vi "AIT 1553 - Parse RT Channels.vi"(6 "Bus Config Info":T10, 7 "FIFO Idx Qs":T12, 8 "error in (no error)":errorcluster, 9 "Bus Page Ref":T1 format="%.0x", 10 "Section GUID":string, 11 "Device Reference in":T1 format="%.0x") -> (0 "error out":errorcluster, 1 "Section BaseRate":u32, 2 "HW Channel - RT Section":T2 {"Message Settings"."Driver Data"."First Word" min=8 max=31; "Message Settings"."Driver Data"."Num Bits" min=1 max=32; "Message Settings"."Driver Data"."Start Bit" min=8 max=31; "Message Settings"."Block Data Refs"."Data Reference" format="%.0x"}, 3 "Device Reference out":T1 format="%.0x")   [LabVIEW 2013, in "AIT 1553 Custom Device.lvlib"]
uses:
  AIT 1553 Custom Device.lvlib
  <vilib>/NI Veristand/Custom Device API/Custom Device Item Ref.ctl
  RT Controls/FIFO Idx Qs.ctl
  RT Controls/AIT 1553 - Board Config Info.ctl
  RT Controls/AIT 1553 - Hardware Type.ctl
  RT Controls/AIT 1553 - RT HW Channel.ctl
  RT Controls/AIT 1553 - Bus Section.ctl
  RT Controls/AIT 1553 - RT Message Settings.ctl
  <vilib>/NI Veristand/Custom Device API/Block Data Reference.ctl
  <vilib>/NI Veristand/Custom Device API/Data Reference.ctl
  RT Controls/AIT 1553 - Driver Data.ctl
  Controls and Global/Start Bit.ctl
  Controls and Global/Number of Bits.ctl
  <vilib>/NI Veristand/Custom Device Tools/Custom Device Utility Library/RT Debug String Color Spec.ctl
  <vilib>/NI Veristand/Custom Device Tools/Custom Device Utility Library/NI VeriStand - Search for Item by GUID.vi
  Controls and Global/Global.vi
  <vilib>/NI Veristand/Custom Device Tools/Custom Device Utility Library/Custom Device Utility Library.lvlib
  <vilib>/NI Veristand/Custom Device API/Custom Device API.lvlib
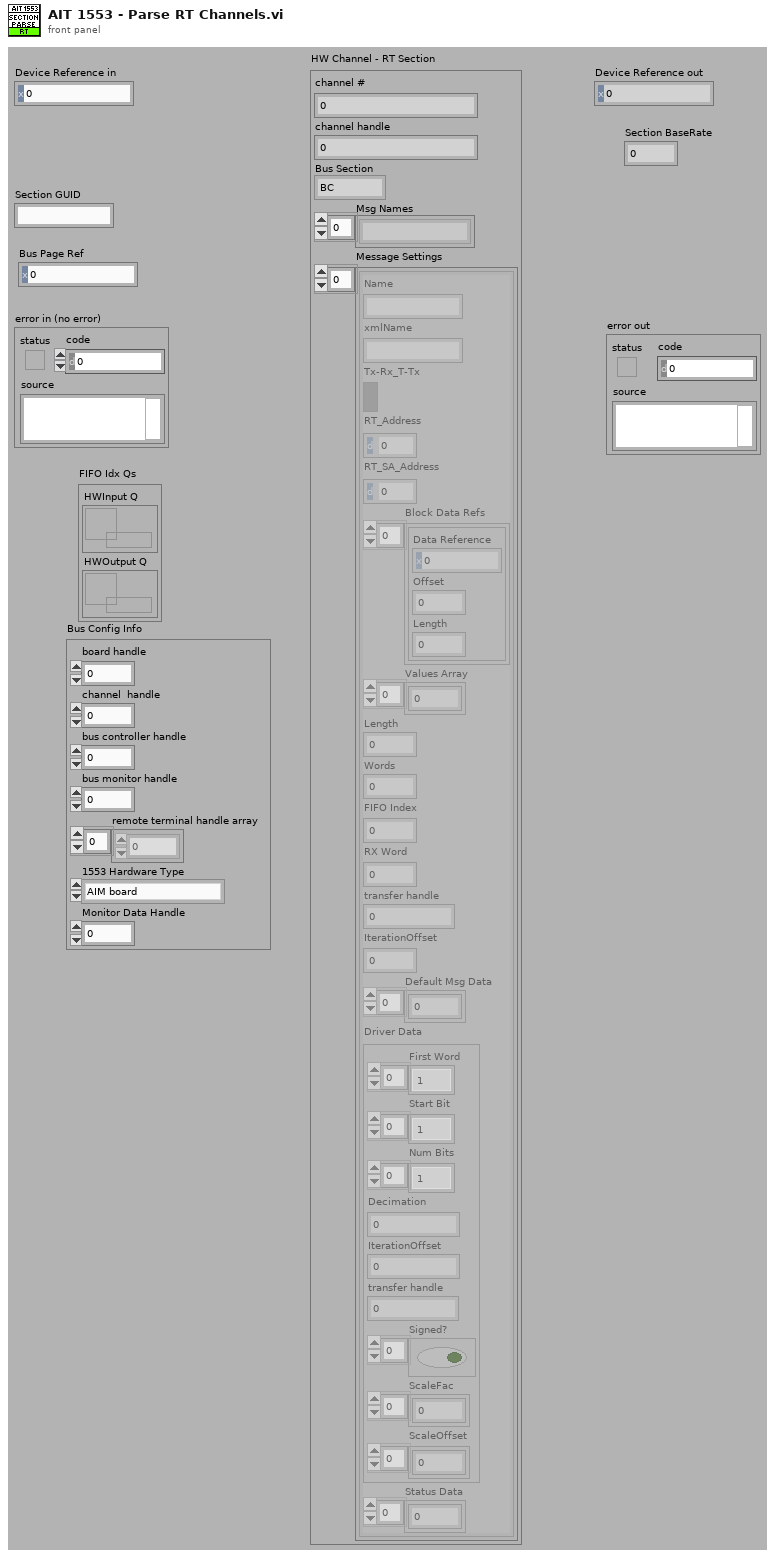
[diagram p1: front panel]
types:
  T1 = typedef "Custom Device API.lvlib/Custom Device Item Ref.ctl" = u64
  T2 = typedef "AIT 1553 Custom Device.lvlib/AIT 1553 - RT HW Channel.ctl" = cluster{"channel #":u16, "channel handle":u32, "Bus Section":T3, "Msg Names":string[], "Message Settings":T4[]}
  T3 = typedef "AIT 1553 Custom Device.lvlib/AIT 1553 - Bus Section.ctl" = enum16{"BC", "BM", "RT"}
  T4 = typedef "AIT 1553 Custom Device.lvlib/AIT 1553 - RT Message Settings.ctl" = cluster{"Name":string, "xmlName":string, "Tx-Rx_T-Tx":bool, "RT_Address":u8, "RT_SA_Address":u8, "Block Data Refs":T5[], "Values Array":dbl[], "Length":i32, "Words":i32, "FIFO Index":i32, "RX Word":u32, "transfer handle":u32, "IterationOffset":i32, "Default Msg Data":u16[], "Driver Data":T7, "Status Data":u32[]}
  T5 = typedef "Custom Device API.lvlib/Block Data Reference.ctl" = cluster{"Data Reference":T6, "Offset":i32, "Length":i32}
  T6 = typedef "Custom Device API.lvlib/Data Reference.ctl" = i32
  T7 = typedef "AIT 1553 Custom Device.lvlib/AIT 1553 - Driver Data.ctl" = cluster{"First Word":T8[], "Start Bit":T8[], "Num Bits":T9[], "Decimation":i32, "IterationOffset":i32, "transfer handle":u32, "Signed?":bool[], "ScaleFac":dbl[], "ScaleOffset":dbl[]}
  T8 = typedef "AIT 1553 Custom Device.lvlib/Start Bit.ctl" = i32
  T9 = typedef "AIT 1553 Custom Device.lvlib/Number of Bits.ctl" = i32
  T10 = typedef "AIT 1553 Custom Device.lvlib/AIT 1553 - Board Config Info.ctl" = cluster{"board handle":u32, "channel  handle":u32, "bus controller handle":u32, "bus monitor handle":u32, "remote terminal handle array":u32[], "1553 Hardware Type":T11, "Monitor Data Handle":u32}
  T11 = typedef "AIT 1553 Custom Device.lvlib/AIT 1553 - Hardware Type.ctl" = enum16{"AIM board", "AIT Board"}
  T12 = typedef "AIT 1553 Custom Device.lvlib/FIFO Idx Qs.ctl" = cluster{"HWInput Q":refnum<queue>, "HWOutput Q":refnum<queue>}
  T13 = typedef "Custom Device Utility Library.lvlib/RT Debug String Color Spec.ctl" = u16
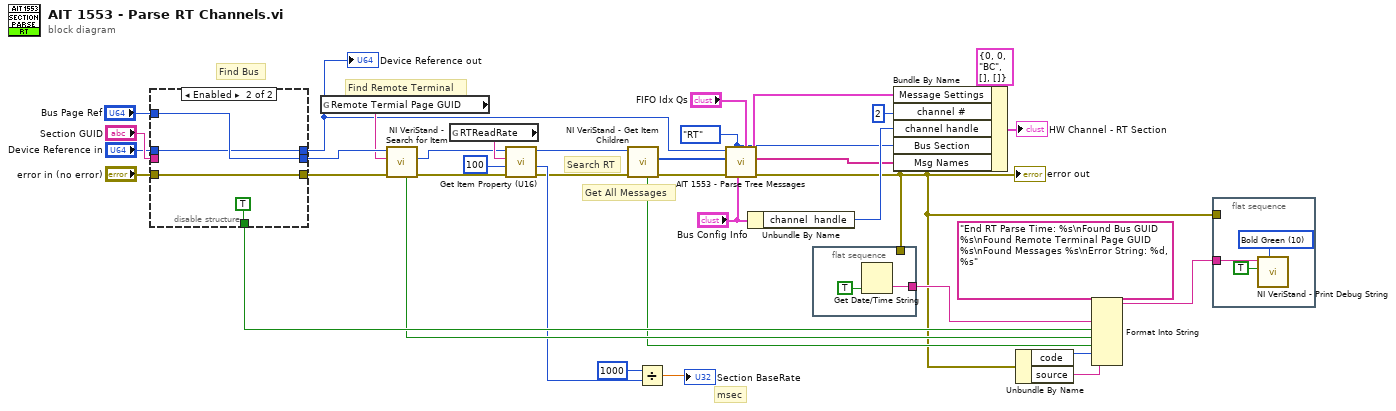
[diagram p0: block diagram]
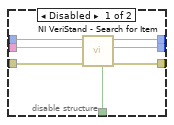
[diagram p2: hidden frame]
diagram:
  w15 = AIT_1553_-_Bus_Section."RT" ("Bus Section")
  # "msec"
  # "Find Remote Terminal"
  # "Find Bus"
  # "Get All Messages"
  # "Search RT"
  n1 = disable-structure shown="Enabled" {
    disable-tunnel: "Section GUID" -> [w44 _]
    disable-tunnel: "Device Reference in" -> [w43 w46]
    disable-tunnel: "error in (no error)" -> [w42 w45]
    disable-tunnel: [w41 w47] -> w28
    disable-tunnel: [w40 w45] -> w27
    disable-tunnel: [w39 TRUE ("Found")] -> w23
    disable-tunnel: [w38 w46] -> w14
    disable-tunnel: "Bus Page Ref" -> [_ w47]
    frame Disabled {
      n2 = call-poly <vilib>:"NI VeriStand - Search for Item.vi"("error in"=w42, "Item GUID"=w44, "Section Ref in"=w43) -> ("error out"=w40:errorcluster, "Item Ref"=w41:T1, "Section Ref out"=w38:T1, "Found"=w39:bool)  [unwired: 5 in]
    }
    frame Enabled {
    }
  }
  "Device Reference out" <- w14
  n3 = global read "Global.vi" "Remote Termial Page GUID"() -> (w26:string)
  n4 = call-poly <vilib>:"NI VeriStand - Search for Item.vi"("error in"=w27, "Item GUID"=w26, "Section Ref in"=w28) -> ("error out"=w7:errorcluster, "Item Ref"=w6:T1, "Found"=w22:bool)  [unwired: 5 in, 1 out]
  n5 = global read "Global.vi" "RTReadRate"() -> (w8:string)
  n6 = call <vilib>:"Get Item Property (U16).vi"("error in (no error)"=w7, "Default Value"=u16 100 ("Section BaseRate"), "Property Name"=w8, "Item Ref in"=w6) -> ("error out"=w3:errorcluster, "Value"=w9:u16, "Item Ref out"=w4:T1)  [unwired: 4 in, 1 out]
  n7 = call <vilib>:"NI VeriStand - Get Item Children.vi"("error in (no error)"=w3, "Item Ref in"=w4) -> ("error out"=w20:errorcluster, "Child Refs"=w34:T1[], "Found"=w18:bool)  [unwired: 6 in, 1 out]
  n8 = Divide(x=u16 1000 ("Section BaseRate"), y=w9) -> (x/y=→"Section BaseRate":dbl)
  n9 = call "AIT 1553 - Parse Tree Messages.vi"("FIFO Idx Qs"="FIFO Idx Qs", "Bus Config Info"="Bus Config Info", "Bus Section"=w15, "error out"=w20, "Message Refs"=w34, "Custom Device Ref"=w14) -> ("error out"=w11:errorcluster, "Msg Names"=w13:string[], "Message Settings"=w31:T4[])  [unwired: 3 in]
  "error out" <- w11
  n10 = Unbundle By Name("Bus Config Info") -> ("channel  handle"=w29:u32)
  n11 = flat-sequence {
    tunnel: [w50] -> w12
    tunnel: w11 -> [_]
    frame #0 {
      n12 = Get Date/Time String(want seconds? (F)=TRUE) -> (time string=w50:string)  [unwired: 2 in, 1 out]
    }
  }
  n13 = Bundle By Name(cluster=T2 {"channel #"=0, "channel handle"=0, "Bus Section"=enum."BC", "Msg Names"=[], "Message Settings"=[]} ("HW Channel"), "Message Settings"=w31, "channel #"=u16 2, "channel handle"=w29, "Bus Section"=w15, "Msg Names"=w13) -> (→"HW Channel - RT Section":T2)
  n14 = Unbundle By Name(w11) -> ("code"=w19:i32, "source"=w25:string)
  n15 = Format Into String(format string="End RT Parse Time: %s\nFound Bus GUID %s\nFound Remote Terminal Page GUID  %s\nFound Messages %s\nError String: %d, %s", w12, w23, w22, w18, w19, w25) -> (resulting string=w24:string)  [unwired: 2 in, 1 out]
  n16 = flat-sequence {
    tunnel: w24 -> [w53]
    tunnel: w11 -> [_]
    frame #0 {
      w52 = T13 10 items=["Plain White"=7, "Bold White"=15, "Bold Blue"=9, "Bold Green"=10, "Bold Red"=12] ("Attribute")
      n17 = call <vilib>:"NI VeriStand - Print Debug String.vi"("Attribute"=w52, "Add to log file? (T)"=TRUE, "Message"=w53) -> ()  [unwired: 8 in, 1 out]
    }
  }
